vi "InitCW.vi"(8 "error in (no error)":errorcluster, 9 "Camera Controller":T1(ring), 10 "SceneGraphDisp":refnum<vi>) -> (0 "error out":errorcluster, 3 "Control Window out":refnum<class "Control Window.lvclass">)   [LabVIEW 2015, in "Control Window.lvclass"]
uses:
  Control Window.lvclass
  Control Window.lvclass/Control Window.ctl
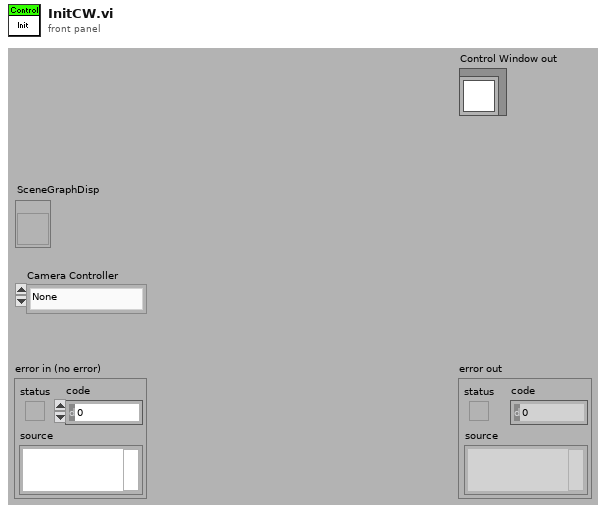
[diagram p1: front panel]
types:
  T1 = enum16{"None", "Spherical", "Flying", "Oriented"}
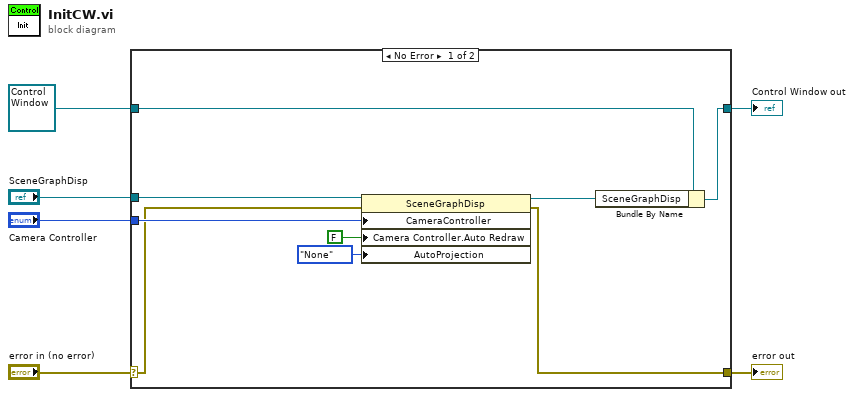
[diagram p0: block diagram]
diagram:
  n1 = case shown="No Error" "error in (no error)" {
    selector: "error in (no error)" -> [w13 w17]
    tunnel: [w9 w17] -> w5
    tunnel: [w11 w16] -> w3
    tunnel: refnum<class "Control Window.lvclass"> refnum ("Control Window in") -> [w12 w16]
    tunnel: "SceneGraphDisp" -> [w15 _]
    tunnel: "Camera Controller" -> [w14 _]
    frame No Error {
      n2 = property class="SceneGraphDisp"(reference=w15, error in=w13, "CameraController"=w14, "Camera Controller.Auto Redraw"=FALSE ("Camera Controller:Auto Redraw"), "AutoProjection"=enum16{"None", "Perspective", "Orthographic"}."None" ("Automatic Projection Mode")) -> (reference out=w10:refnum<vi>, error out=w9:errorcluster)
      n3 = Bundle By Name(cluster=w12, "SceneGraphDisp"=w10) -> (w11:refnum<class "Control Window.lvclass">)
    }
    frame Error {
    }
  }
  "error out" <- w5
  "Control Window out" <- w3
